vi "Drive_8CANSwerve.vi"(0 "FrontLeftRotation":dbl, 1 "FrontLeftDrive":dbl, 2 "FrontRightRotation":dbl, 3 "FrontRightDrive":dbl, 4 "RearLeftRotation":dbl, 5 "RearLeftDrive":dbl, 6 "RearRightRotation":dbl, 7 "RearRightDrive":dbl, 11 "PIDInputs":T6, 15 "RotationSettings":T5={"T0"=0, "Mode"=enum."Calibrate", "Rotation Neutral Mode"=enum."Override to Coast", "Rotation Control Mode"=0, "Feedback Device"=8} {"Rotation Control Mode" items=["PercentOutput"=0, "Position"=1, "Velocity"=2, "Current"=3, "Follower"=5, "MotionProfile"=6, "MotionMagic"=7, "MotionProfileArc"=10, "Disabled"=15]; "Feedback Device" items=["QuadEncoder"=0, "Analog"=2, "Tachometer"=4, "Pulse Width Encoded Position"=8, "Sensor Sum (S0 + S1)"=9, "Sensor Difference (D0 - D1)"=10, "Remote Source 0"=11, "Remote Source 1"=12, "Software Emulated"=15]}) -> ()   [LabVIEW 2018]
uses:
  SwerveRotationCalibrate.ctl
  <vilib>/Rock Robotics/WPI/ThirdParty/Phoenix-LabVIEW/Motor Controller/Controls/CTRE_Phoenix_MotorControl_NeutralMode.ctl
  <vilib>/Rock Robotics/WPI/ThirdParty/Phoenix-LabVIEW/Motor Controller/Controls/CTRE_Phoenix_MotorControl_ControlMode.ctl
  <vilib>/Rock Robotics/WPI/ThirdParty/Phoenix-LabVIEW/Motor Controller/Controls/CTRE_Phoenix_MotorControl_FeedbackDevice.ctl
  <vilib>/Rock Robotics/WPI/ThirdParty/REV Robotics/SPARK MAX/Typedef/Spark MAX Control Type.ctl
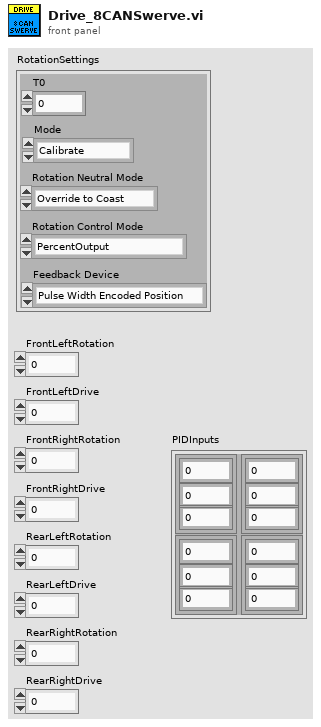
[diagram p1: front panel]
types:
  T1 = typedef "SwerveRotationCalibrate.ctl" = enum16{"Calibrate", "Home", "ManualHome", "ResetQuad", "Drive"}
  T2 = typedef "CTRE_Phoenix_MotorControl_NeutralMode.ctl" = enum8{"EEPROMSetting", "Override to Coast", "Override to Brake"}
  T3 = typedef "CTRE_Phoenix_MotorControl_ControlMode.ctl" = u16
  T4 = typedef "CTRE_Phoenix_MotorControl_FeedbackDevice.ctl" = i8
  T5 = cluster{"T0":u32, "Mode":T1, "Rotation Neutral Mode":T2, "Rotation Control Mode":T3, "Feedback Device":T4}
  T6 = cluster{"Motor1":cluster{"P":dbl, "I":dbl, "D":dbl}, "Motor3":cluster{"P":dbl, "I":dbl, "D":dbl}, "Motor2":cluster{"P":dbl, "I":dbl, "D":dbl}, "Motor4":cluster{"P":dbl, "I":dbl, "D":dbl}}
  T7 = typedef "Spark MAX Control Type.ctl" = enum16{"Percent VBus", "Voltage", "Velocity", "Position", "Smart Motion", "Current", "Smart Velocity"}
  T8 = typedef "WPI_MotorControlDeviceRef.ctl" = cluster{"DeviceStatus":errorcluster, "Type":T9, "PWM":cluster{"PWM Channel":T10, "DeadBand":T11}, "CAN":cluster{"Device Number":u8, "SetOutput VI Ref":variant, "GetOutput VI Ref":variant, "Enable VI Ref":variant, "Disable VI Ref":variant, "Data":variant}, "Invert":bool, "DIO PWM":cluster{"PWM \"Enable\" Channel":T10, "DIOChannel":T12, "PWM Rate":dbl}}
  T9 = typedef "WPI_MotorControlType.ctl" = enum16{"PWM", "CAN", "DIO PWM"}
  T10 = typedef "FPGA_DIOPWMChannel.ctl" = enum8{"PWM 0", "PWM 1", "PWM 2", "PWM 3", "PWM 4", "PWM 5", "PWM 6", "PWM 7", "PWM 8", "PWM 9", "PWM MXP 0", "PWM MXP 1", "PWM MXP 2", "PWM MXP 3", "PWM MXP 4", "PWM MXP 5", "PWM MXP 6", "PWM MXP 7", "PWM MXP 8", "PWM MXP 9", "Invalid"}
  T11 = typedef "WPI_PWMDeadband.ctl" = cluster{"Name":string, "maxPositivePwm":i32, "minPositivePwm":i32, "centerPwm":i32, "maxNegativePwm":i32, "minNegativePwm":i32, "angularRange":u16}
  T12 = typedef "FPGA_DIOChannel.ctl" = enum8{"DIO 0", "DIO 1", "DIO 2", "DIO 3", "DIO 4", "DIO 5", "DIO 6", "DIO 7", "DIO 8", "DIO 9", "DIO MXP 0", "DIO MXP 1", "DIO MXP 2", "DIO MXP 3", "DIO MXP 4", "DIO MXP 5", "DIO MXP 6", "DIO MXP 7", "DIO MXP 8", "DIO MXP 9", "DIO MXP 10", "DIO MXP 11", "DIO MXP 12", "DIO MXP 13", "DIO MXP 14", "DIO MXP 15", "SPI Port CS1", "SPI Port CS2", "SPI Port CS3", "SPI Port MISO", "SPI Port MOSI", "Invalid"}
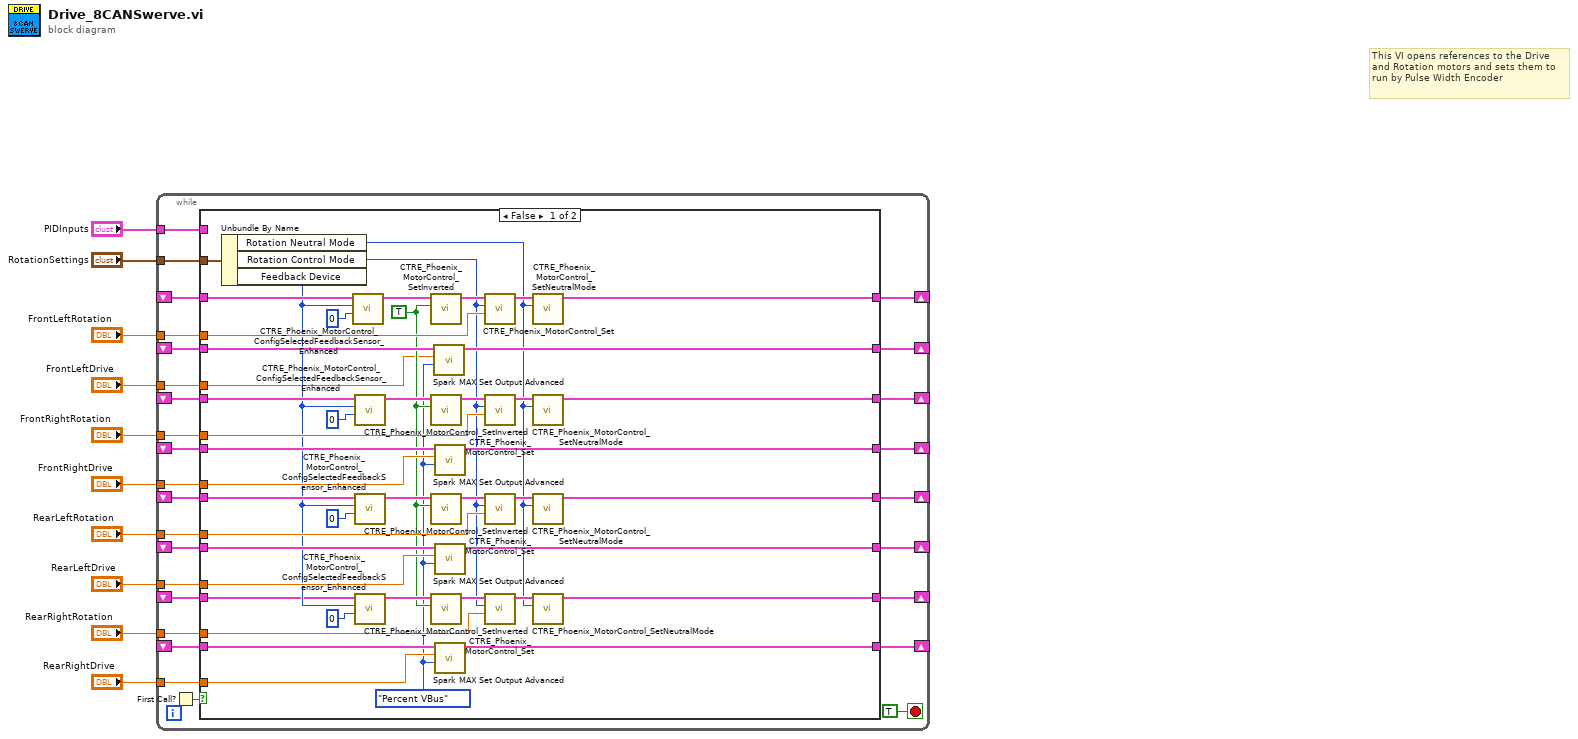
[diagram p0: block diagram]
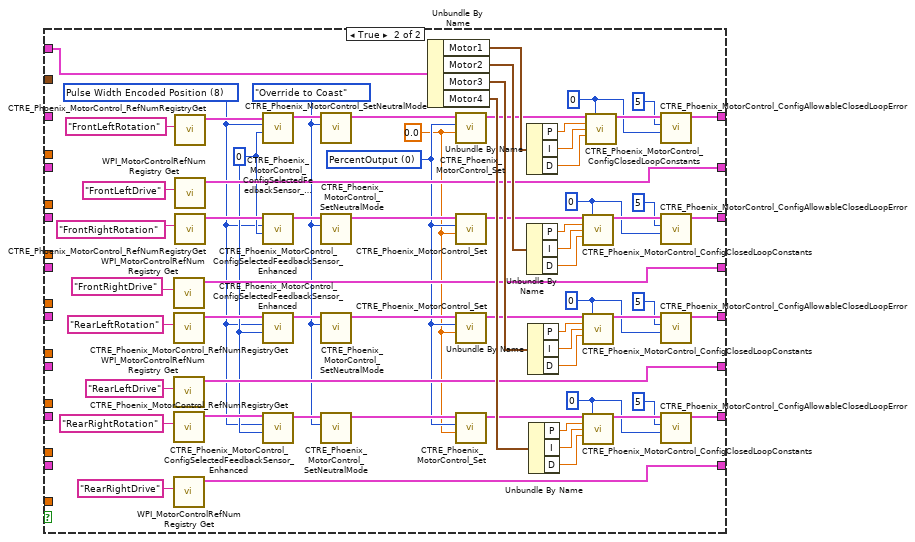
[diagram p2: hidden frame]
diagram:
  # "This VI opens references to the Drive and Rotation motors and sets them to run by Pulse Width Encoder"
  n1 = while {
    shift-right: [w38] -> _
    shift-left: _ -> [w37]
    shift-right: [w15] -> _
    shift-left: _ -> [w35]
    shift-right: [w11] -> _
    shift-left: _ -> [w34]
    shift-right: [w14] -> _
    shift-left: _ -> [w33]
    shift-right: [w36] -> _
    shift-left: _ -> [w32]
    shift-right: [w13] -> _
    shift-left: _ -> [w31]
    shift-right: [w16] -> _
    shift-left: _ -> [w30]
    shift-right: [w12] -> _
    shift-left: _ -> [w29]
    tunnel: "FrontLeftRotation" -> [w26]
    tunnel: "FrontLeftDrive" -> [w25]
    tunnel: "FrontRightRotation" -> [w24]
    tunnel: "FrontRightDrive" -> [w23]
    tunnel: "RearLeftRotation" -> [w22]
    tunnel: "RearLeftDrive" -> [w21]
    tunnel: "RearRightRotation" -> [w20]
    tunnel: "RearRightDrive" -> [w19]
    tunnel: "PIDInputs" -> [w18]
    tunnel: "RotationSettings" -> [w17]
    stop <- TRUE stop-if-true
    n2 = First Call?() -> (First Call?: T/F=w27:bool)
    n3 = case shown="False" w27 {
      tunnel: [w52 w94] -> w38
      tunnel: w37 -> [w67 _]
      tunnel: [w77 w125] -> w15
      tunnel: [w50 w85] -> w11
      tunnel: [w76 w123] -> w14
      tunnel: [w48 w96] -> w36
      tunnel: [w75 w121] -> w13
      tunnel: [w46 w99] -> w16
      tunnel: [w74 w119] -> w12
      tunnel: w35 -> [w68 _]
      tunnel: w34 -> [w69 _]
      tunnel: w33 -> [w66 _]
      tunnel: w32 -> [w65 _]
      tunnel: w31 -> [w64 _]
      tunnel: w30 -> [w41 _]
      tunnel: w29 -> [w63 _]
      tunnel: w26 -> [w84 _]
      tunnel: w25 -> [w39 _]
      tunnel: w24 -> [w83 _]
      tunnel: w23 -> [w82 _]
      tunnel: w22 -> [w81 _]
      tunnel: w21 -> [w80 _]
      tunnel: w20 -> [w79 _]
      tunnel: w19 -> [w78 _]
      tunnel: w18 -> [_ w142]
      tunnel: w17 -> [w42 _]
      frame False {
        w40 = Spark_MAX_Control_Type."Percent VBus" ("Control Mode")
        w57 = TRUE
        n4 = Unbundle By Name(w42) -> ("Rotation Neutral Mode"=w43:T2, "Rotation Control Mode"=w44:T3, "Feedback Device"=w45:T4)
        n5 = call <vilib>:"CTRE_Phoenix_MotorControl_ConfigSelectedFeedbackSensor_Enhanced.vi"("pidLoopIdx"=0, "Feedback Device"=w45, "PhoenixMotorControlDevRef"=w67) -> ("PhoenixMotorControlDevRef"=w59:T8)  [unwired: 7 in, 1 out]
        n6 = call <vilib>:"CTRE_Phoenix_MotorControl_ConfigSelectedFeedbackSensor_Enhanced.vi"("pidLoopIdx"=0, "Feedback Device"=w45, "PhoenixMotorControlDevRef"=w69) -> ("PhoenixMotorControlDevRef"=w60:T8)  [unwired: 7 in, 1 out]
        n7 = call <vilib>:"CTRE_Phoenix_MotorControl_ConfigSelectedFeedbackSensor_Enhanced.vi"("pidLoopIdx"=0, "Feedback Device"=w45, "PhoenixMotorControlDevRef"=w65) -> ("PhoenixMotorControlDevRef"=w61:T8)  [unwired: 7 in, 1 out]
        n8 = call <vilib>:"CTRE_Phoenix_MotorControl_ConfigSelectedFeedbackSensor_Enhanced.vi"("pidLoopIdx"=0, "Feedback Device"=w45, "PhoenixMotorControlDevRef"=w41) -> ("PhoenixMotorControlDevRef"=w62:T8)  [unwired: 7 in, 1 out]
        n9 = call <vilib>:"CTRE_Phoenix_MotorControl_SetInverted.vi"("Invert?"=w57, "PhoenixMotorControlDevRef"=w59) -> ("PhoenixMotorControlDevRef"=w58:T8)  [unwired: 8 in, 1 out]
        n10 = call <vilib>:"CTRE_Phoenix_MotorControl_SetInverted.vi"("Invert?"=w57, "PhoenixMotorControlDevRef"=w60) -> ("PhoenixMotorControlDevRef"=w54:T8)  [unwired: 8 in, 1 out]
        n11 = call <vilib>:"CTRE_Phoenix_MotorControl_SetInverted.vi"("Invert?"=w57, "PhoenixMotorControlDevRef"=w61) -> ("PhoenixMotorControlDevRef"=w55:T8)  [unwired: 8 in, 1 out]
        n12 = call <vilib>:"CTRE_Phoenix_MotorControl_SetInverted.vi"("Invert?"=w57, "PhoenixMotorControlDevRef"=w62) -> ("PhoenixMotorControlDevRef"=w56:T8)  [unwired: 8 in, 1 out]
        n13 = call <vilib>:"Spark MAX Set Output Advanced.vi"("Control Mode"=w40, "Setpoint"=w39, "MotorControlDevRef"=w68) -> ("MotorControlDevRef"=w77:T8)  [unwired: 7 in, 1 out]
        n14 = call <vilib>:"Spark MAX Set Output Advanced.vi"("Control Mode"=w40, "Setpoint"=w82, "MotorControlDevRef"=w66) -> ("MotorControlDevRef"=w76:T8)  [unwired: 7 in, 1 out]
        n15 = call <vilib>:"Spark MAX Set Output Advanced.vi"("Control Mode"=w40, "Setpoint"=w80, "MotorControlDevRef"=w64) -> ("MotorControlDevRef"=w75:T8)  [unwired: 7 in, 1 out]
        n16 = call <vilib>:"Spark MAX Set Output Advanced.vi"("Control Mode"=w40, "Setpoint"=w78, "MotorControlDevRef"=w63) -> ("MotorControlDevRef"=w74:T8)  [unwired: 7 in, 1 out]
        n17 = call <vilib>:"CTRE_Phoenix_MotorControl_Set.vi"("Output"=w84, "Control Mode"=w44, "PhoenixMotorControlDevRef"=w58) -> ("PhoenixMotorControlDevRef"=w53:T8)  [unwired: 7 in, 1 out]
        n18 = call <vilib>:"CTRE_Phoenix_MotorControl_Set.vi"("Output"=w83, "Control Mode"=w44, "PhoenixMotorControlDevRef"=w54) -> ("PhoenixMotorControlDevRef"=w51:T8)  [unwired: 7 in, 1 out]
        n19 = call <vilib>:"CTRE_Phoenix_MotorControl_Set.vi"("Output"=w81, "Control Mode"=w44, "PhoenixMotorControlDevRef"=w55) -> ("PhoenixMotorControlDevRef"=w49:T8)  [unwired: 7 in, 1 out]
        n20 = call <vilib>:"CTRE_Phoenix_MotorControl_Set.vi"("Output"=w79, "Control Mode"=w44, "PhoenixMotorControlDevRef"=w56) -> ("PhoenixMotorControlDevRef"=w47:T8)  [unwired: 7 in, 1 out]
        n21 = call <vilib>:"CTRE_Phoenix_MotorControl_SetNeutralMode.vi"("Motor Control Neutral Mode"=w43, "PhoenixMotorControlDevRef"=w53) -> ("PhoenixMotorControlDevRef"=w52:T8)  [unwired: 8 in, 1 out]
        n22 = call <vilib>:"CTRE_Phoenix_MotorControl_SetNeutralMode.vi"("Motor Control Neutral Mode"=w43, "PhoenixMotorControlDevRef"=w51) -> ("PhoenixMotorControlDevRef"=w50:T8)  [unwired: 8 in, 1 out]
        n23 = call <vilib>:"CTRE_Phoenix_MotorControl_SetNeutralMode.vi"("Motor Control Neutral Mode"=w43, "PhoenixMotorControlDevRef"=w49) -> ("PhoenixMotorControlDevRef"=w48:T8)  [unwired: 8 in, 1 out]
        n24 = call <vilib>:"CTRE_Phoenix_MotorControl_SetNeutralMode.vi"("Motor Control Neutral Mode"=w43, "PhoenixMotorControlDevRef"=w47) -> ("PhoenixMotorControlDevRef"=w46:T8)  [unwired: 8 in, 1 out]
      }
      frame True {
        w101 = 0.0 ("Output")
        w102 = T3 0 items=["PercentOutput"=0, "Position"=1, "Velocity"=2, "Current"=3, "Follower"=5, "MotionProfile"=6, "MotionMagic"=7, "MotionProfileArc"=10, "Disabled"=15] ("Control Mode")
        w111 = CTRE_Phoenix_MotorControl_NeutralMode."Override to Coast" ("Motor Control Neutral Mode")
        w116 = T4 8 items=["QuadEncoder"=0, "Analog"=2, "Tachometer"=4, "Pulse Width Encoded Position"=8, "Sensor Sum (S0 + S1)"=9, "Sensor Difference (D0 - D1)"=10, "Remote Source 0"=11, "Remote Source 1"=12, "Software Emulated"=15] ("Feedback Device")
        w117 = 0 ("pidLoopIdx")
        w98 = 0 ("slotIdx")
        w88 = 0 ("slotIdx")
        w87 = 0 ("slotIdx")
        w86 = 0 ("slotIdx")
        n25 = call <vilib>:"WPI_MotorControlRefNum Registry Get.vi"("refnum name"="FrontRightDrive") -> ("MotorControlDevRef"=w123:T8)  [unwired: 9 in, 1 out]
        n26 = call <vilib>:"CTRE_Phoenix_MotorControl_RefNumRegistryGet.vi"("refnum name"="RearLeftRotation") -> ("PhoenixMotorControlDevRef"=w122:T8)  [unwired: 9 in, 1 out]
        n27 = call <vilib>:"WPI_MotorControlRefNum Registry Get.vi"("refnum name"="RearLeftDrive") -> ("MotorControlDevRef"=w121:T8)  [unwired: 9 in, 1 out]
        n28 = call <vilib>:"CTRE_Phoenix_MotorControl_RefNumRegistryGet.vi"("refnum name"="RearRightRotation") -> ("PhoenixMotorControlDevRef"=w120:T8)  [unwired: 9 in, 1 out]
        n29 = call <vilib>:"WPI_MotorControlRefNum Registry Get.vi"("refnum name"="RearRightDrive") -> ("MotorControlDevRef"=w119:T8)  [unwired: 9 in, 1 out]
        n30 = call <vilib>:"CTRE_Phoenix_MotorControl_RefNumRegistryGet.vi"("refnum name"="FrontLeftRotation") -> ("PhoenixMotorControlDevRef"=w126:T8)  [unwired: 9 in, 1 out]
        n31 = call <vilib>:"WPI_MotorControlRefNum Registry Get.vi"("refnum name"="FrontLeftDrive") -> ("MotorControlDevRef"=w125:T8)  [unwired: 9 in, 1 out]
        n32 = call <vilib>:"CTRE_Phoenix_MotorControl_RefNumRegistryGet.vi"("refnum name"="FrontRightRotation") -> ("PhoenixMotorControlDevRef"=w124:T8)  [unwired: 9 in, 1 out]
        n33 = call <vilib>:"CTRE_Phoenix_MotorControl_ConfigSelectedFeedbackSensor_Enhanced.vi"("pidLoopIdx"=w117, "Feedback Device"=w116, "PhoenixMotorControlDevRef"=w126) -> ("PhoenixMotorControlDevRef"=w115:T8)  [unwired: 7 in, 1 out]
        n34 = call <vilib>:"CTRE_Phoenix_MotorControl_ConfigSelectedFeedbackSensor_Enhanced.vi"("pidLoopIdx"=w117, "Feedback Device"=w116, "PhoenixMotorControlDevRef"=w124) -> ("PhoenixMotorControlDevRef"=w113:T8)  [unwired: 7 in, 1 out]
        n35 = call <vilib>:"CTRE_Phoenix_MotorControl_ConfigSelectedFeedbackSensor_Enhanced.vi"("pidLoopIdx"=w117, "Feedback Device"=w116, "PhoenixMotorControlDevRef"=w122) -> ("PhoenixMotorControlDevRef"=w114:T8)  [unwired: 7 in, 1 out]
        n36 = call <vilib>:"CTRE_Phoenix_MotorControl_ConfigSelectedFeedbackSensor_Enhanced.vi"("pidLoopIdx"=w117, "Feedback Device"=w116, "PhoenixMotorControlDevRef"=w120) -> ("PhoenixMotorControlDevRef"=w112:T8)  [unwired: 7 in, 1 out]
        n37 = call <vilib>:"CTRE_Phoenix_MotorControl_SetNeutralMode.vi"("Motor Control Neutral Mode"=w111, "PhoenixMotorControlDevRef"=w115) -> ("PhoenixMotorControlDevRef"=w108:T8)  [unwired: 8 in, 1 out]
        n38 = call <vilib>:"CTRE_Phoenix_MotorControl_SetNeutralMode.vi"("Motor Control Neutral Mode"=w111, "PhoenixMotorControlDevRef"=w113) -> ("PhoenixMotorControlDevRef"=w106:T8)  [unwired: 8 in, 1 out]
        n39 = call <vilib>:"CTRE_Phoenix_MotorControl_SetNeutralMode.vi"("Motor Control Neutral Mode"=w111, "PhoenixMotorControlDevRef"=w114) -> ("PhoenixMotorControlDevRef"=w104:T8)  [unwired: 8 in, 1 out]
        n40 = call <vilib>:"CTRE_Phoenix_MotorControl_SetNeutralMode.vi"("Motor Control Neutral Mode"=w111, "PhoenixMotorControlDevRef"=w112) -> ("PhoenixMotorControlDevRef"=w110:T8)  [unwired: 8 in, 1 out]
        n41 = Unbundle By Name(w142) -> ("Motor1"=w141:cluster{"P":dbl, "I":dbl, "D":dbl}, "Motor2"=w138:cluster{"P":dbl, "I":dbl, "D":dbl}, "Motor3"=w134:cluster{"P":dbl, "I":dbl, "D":dbl}, "Motor4"=w130:cluster{"P":dbl, "I":dbl, "D":dbl})
        n42 = call <vilib>:"CTRE_Phoenix_MotorControl_Set.vi"("Output"=w101, "Control Mode"=w102, "PhoenixMotorControlDevRef"=w108) -> ("PhoenixMotorControlDevRef"=w107:T8)  [unwired: 7 in, 1 out]
        n43 = call <vilib>:"CTRE_Phoenix_MotorControl_Set.vi"("Output"=w101, "Control Mode"=w102, "PhoenixMotorControlDevRef"=w106) -> ("PhoenixMotorControlDevRef"=w105:T8)  [unwired: 7 in, 1 out]
        n44 = call <vilib>:"CTRE_Phoenix_MotorControl_Set.vi"("Output"=w101, "Control Mode"=w102, "PhoenixMotorControlDevRef"=w104) -> ("PhoenixMotorControlDevRef"=w103:T8)  [unwired: 7 in, 1 out]
        n45 = call <vilib>:"CTRE_Phoenix_MotorControl_Set.vi"("Output"=w101, "Control Mode"=w102, "PhoenixMotorControlDevRef"=w110) -> ("PhoenixMotorControlDevRef"=w109:T8)  [unwired: 7 in, 1 out]
        n46 = Unbundle By Name(w141) -> ("P"=w118:dbl, "I"=w140:dbl, "D"=w139:dbl)
        n47 = Unbundle By Name(w138) -> ("P"=w137:dbl, "I"=w136:dbl, "D"=w135:dbl)
        n48 = Unbundle By Name(w134) -> ("P"=w133:dbl, "I"=w132:dbl, "D"=w131:dbl)
        n49 = Unbundle By Name(w130) -> ("P"=w129:dbl, "I"=w128:dbl, "D"=w127:dbl)
        n50 = call <vilib>:"CTRE_Phoenix_MotorControl_ConfigClosedLoopConstants.vi"("PhoenixMotorControlDevRef"=w105, "slotIdx"=w87, "P"=w137, "I"=w136, "D"=w135) -> ("PhoenixMotorControlDevRef"=w92:T8)  [unwired: 9 in, 1 out]
        n51 = call <vilib>:"CTRE_Phoenix_MotorControl_ConfigClosedLoopConstants.vi"("PhoenixMotorControlDevRef"=w103, "slotIdx"=w88, "P"=w133, "I"=w132, "D"=w131) -> ("PhoenixMotorControlDevRef"=w93:T8)  [unwired: 9 in, 1 out]
        n52 = call <vilib>:"CTRE_Phoenix_MotorControl_ConfigClosedLoopConstants.vi"("PhoenixMotorControlDevRef"=w109, "slotIdx"=w98, "P"=w129, "I"=w128, "D"=w127) -> ("PhoenixMotorControlDevRef"=w100:T8)  [unwired: 9 in, 1 out]
        n53 = call <vilib>:"CTRE_Phoenix_MotorControl_ConfigClosedLoopConstants.vi"("PhoenixMotorControlDevRef"=w107, "slotIdx"=w86, "P"=w118, "I"=w140, "D"=w139) -> ("PhoenixMotorControlDevRef"=w95:T8)  [unwired: 9 in, 1 out]
        n54 = call <vilib>:"CTRE_Phoenix_MotorControl_ConfigAllowableClosedLoopError.vi"("slotIdx"=w86, "allowableClosedLoopError"=5, "PhoenixMotorControlDevRef"=w95) -> ("PhoenixMotorControlDevRef"=w94:T8)  [unwired: 7 in, 1 out]
        n55 = call <vilib>:"CTRE_Phoenix_MotorControl_ConfigAllowableClosedLoopError.vi"("slotIdx"=w87, "allowableClosedLoopError"=5, "PhoenixMotorControlDevRef"=w92) -> ("PhoenixMotorControlDevRef"=w85:T8)  [unwired: 7 in, 1 out]
        n56 = call <vilib>:"CTRE_Phoenix_MotorControl_ConfigAllowableClosedLoopError.vi"("slotIdx"=w88, "allowableClosedLoopError"=5, "PhoenixMotorControlDevRef"=w93) -> ("PhoenixMotorControlDevRef"=w96:T8)  [unwired: 7 in, 1 out]
        n57 = call <vilib>:"CTRE_Phoenix_MotorControl_ConfigAllowableClosedLoopError.vi"("slotIdx"=w98, "allowableClosedLoopError"=5, "PhoenixMotorControlDevRef"=w100) -> ("PhoenixMotorControlDevRef"=w99:T8)  [unwired: 7 in, 1 out]
      }
    }
  }
